vi "dynamic mapping.vi"(8 "error in":errorcluster, 10 "channels available":refnum<class "TBM channel.lvclass">[](array[class]), 11 "module configuration in":refnum<class "TBM module configuration.lvclass">) -> (0 "error out":errorcluster, 2 "reservations":T1[](array[typedef]), 3 "module configuration out":refnum<class "TBM module configuration.lvclass">)   [LabVIEW 2013, in "TBM module configuration.lvclass"]
doc: "Provides an interface for dynamically mapping data at runtime instead of static mapping. For example, a module may which to log all data in a given execution system to disk. In this case, it would register to read data from all groups defined as inputs to the system. Calling code is responsible for providing this data to the requesting component. There is no way to \"undo\" reservations within a component without directly manipulating the component's data. All operations in this module should assume fully qualified channels as input."
uses:
  TBM module configuration.lvclass
  channel/TBM channel.lvclass
  channel reservation.ctl
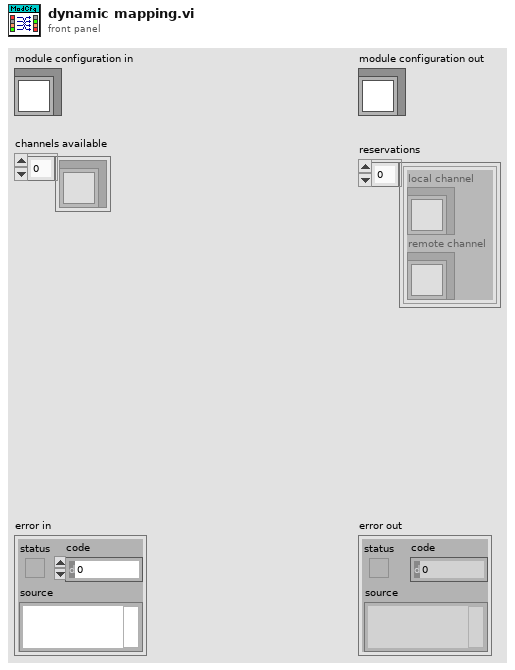
[diagram p1: front panel]
types:
  T1 = typedef "TBM module configuration.lvclass/channel reservation.ctl" = cluster{"local channel":refnum<class "TBM channel.lvclass">, "remote channel":refnum<class "TBM channel.lvclass">}
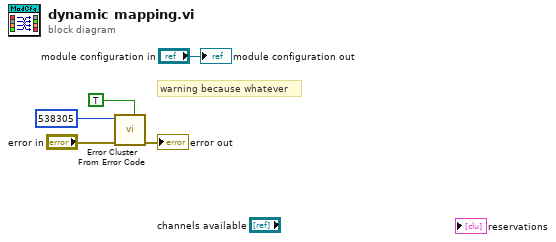
[diagram p0: block diagram]
diagram:
  # "warning because whatever"
  n1 = call <vilib>:"Error Cluster From Error Code.vi"("is warning? (False)"=TRUE, "error in (no error)"="error in", "error code (0)"=538305) -> ("error out"=→"error out":errorcluster)  [unwired: 6 in]
  "module configuration out" <- "module configuration in"
